vi "24_2.vi"() -> ()   [LabVIEW 2020]
uses:
  b6220058-4329-4b3d-852f-7dafbc0d4870.vi
panel:
  out "x-y":u32
  in  "Days":i32=100
  out "size":i32
  in  "Switch":bool
  in  "Input":string="nwneswnwnwsenwnwnwnwnwnwnwnwnwnenwnwnwnw\nseseswswseseswsesenwnwseseswsese\nswneeweneeneneeneeeeeneeeene\neswswnwswswwnwswswswswewswswswswswsw\nwwseneseeneseswwwseneseseneswseswese\nseseseswseseseseswnwswswneseseswsesesese\nnwnewwwwwswnwnwww\nneesenwwswseswswswnwsenwsesewseeeswse\nsweeneesweeswnweewseeneeneneswnw\nswseswseswswseseswseneswseswswsesesesese\nswneneneenenenenenenenenenenenwne\nswswswswswswswswswswswesenwseswswswse\nneeeenweneeneswene\nswwnenwsewwwswswwswwswweewwswwnw\nenewwnenwnenenenwnewnenenwnenenenwee\nnwwnwnwnwnwnwnwenewnwsenwwwwwnwswnw\neeenweeeesweeeneeseeeeswee\nwswwswseswwswswwwnww\nswenwwn..."
  in  "Input Test":string="sesenwnenenewseeswwswswwnenewsewsw\nneeenesenwnwwswnenewnwwsewnenwseswesw\nseswneswswsenwwnwse\nnwnwneseeswswnenewneswwnewseswneseene\nswweswneswnenwsewnwneneseenw\neesenwseswswnenwswnwnwsewwnwsene\nsewnenenenesenwsewnenwwwse\nwenwwweseeeweswwwnwwe\nwsweesenenewnwwnwsenewsenwwsesesenwne\nneeswseenwwswnwswswnw\nnenwswwsewswnenenewsenwsenwnesesenew\nenewnwewneswsewnwswenweswnenwsenwsw\nsweneswneswneneenwnewenewwneswswnese\nswwesenesewenwneswnwwneseswwne\nenesenwswwswneneswsenwnewswseenwsese\nwnwnesenesenenwwnenwsewesewsesesew\nnenewswnwewswnenesenwnesewesw\neneswnwswnwsenenwnwnwwseeswneewsenese\nneswnwewnwnwseenwseesewsenwsweewe\nwseweeenwnesenwwwswnew"
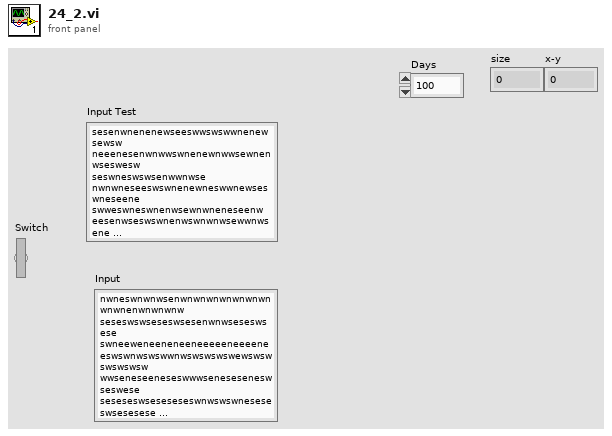
[diagram p1: front panel]
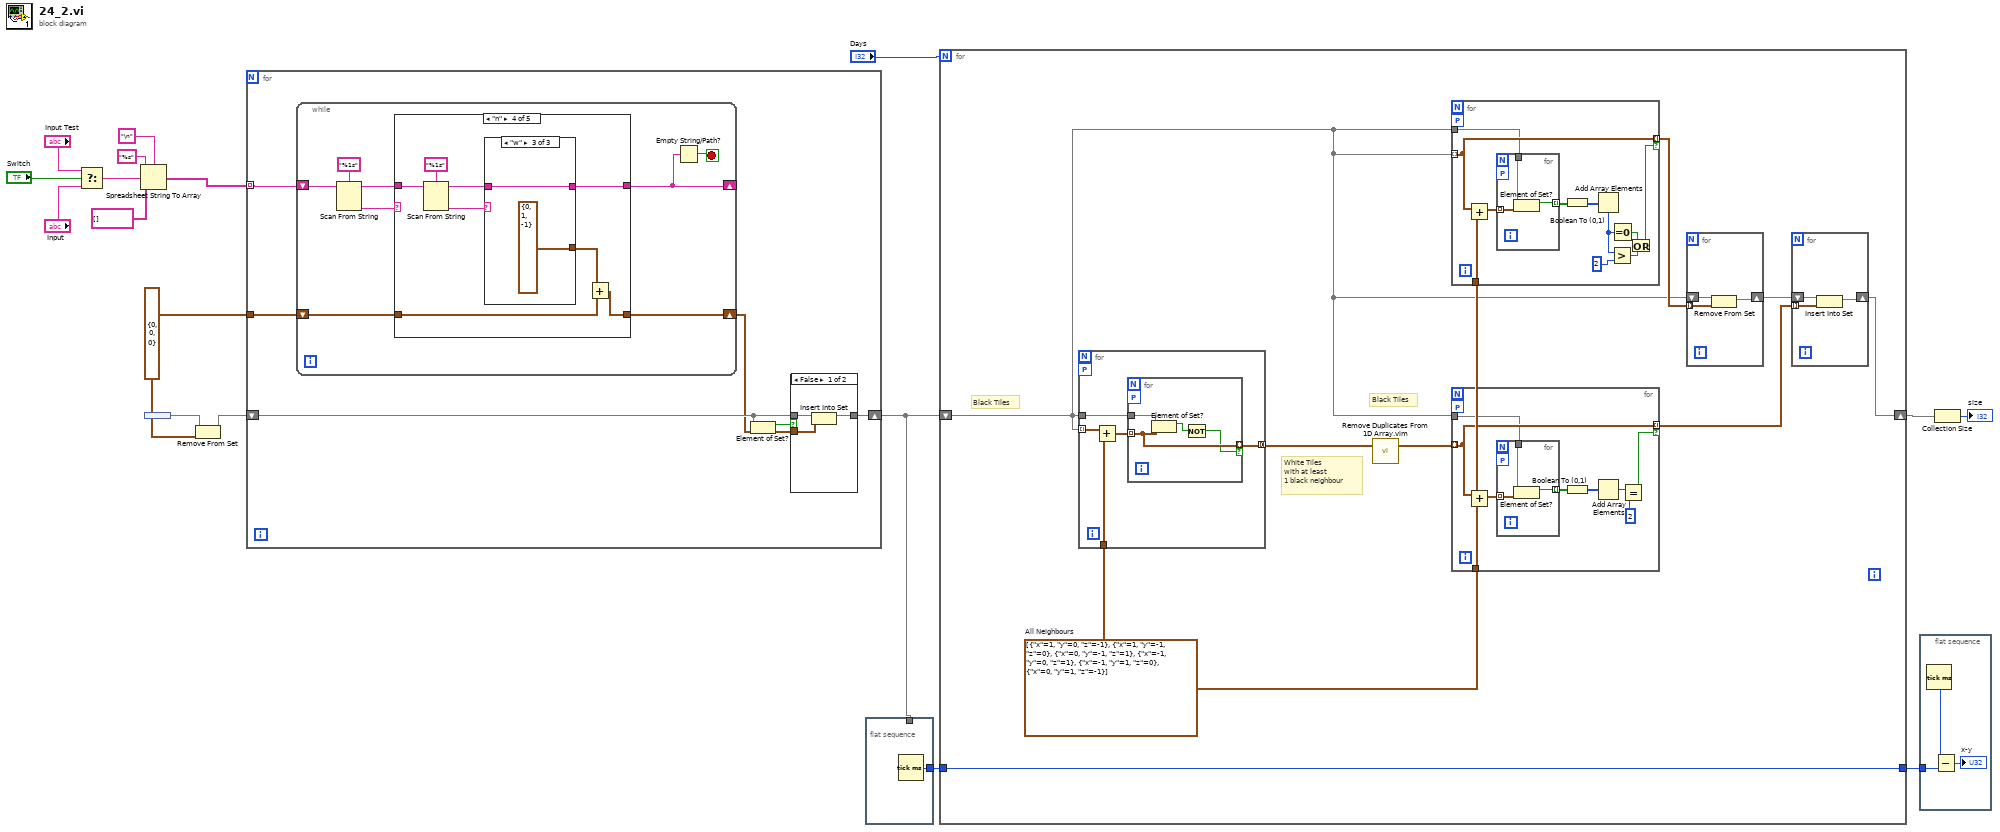
[diagram p0: block diagram]
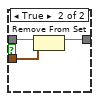
[diagram p2: hidden frame]
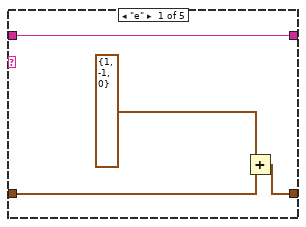
[diagram p3: hidden frame]
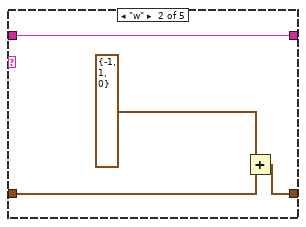
[diagram p4: hidden frame]
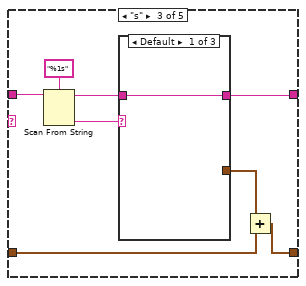
[diagram p5: hidden frame]
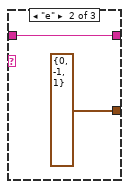
[diagram p6: hidden frame]
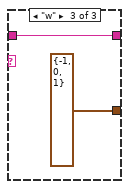
[diagram p7: hidden frame]
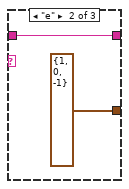
[diagram p9: hidden frame]
diagram:
  w7 = cluster{"x":i32, "y":i32, "z":i32} {"x"=0, "y"=0, "z"=0}
  n1 = Select(t="Input Test", s="Switch", f="Input") -> (s? t:f=w14:string)
  n2 = Spreadsheet String To Array(delimiter (Tab)="\n", format string="%s", spreadsheet string=w14, array type (2D Dbl)=string[] []) -> (array=w10:string[])
  n3 = node(w7) -> (w9:set{cluster{"x":i32, "y":i32, "z":i32}})
  n4 = Remove From Set(10:w7, 11:w9) -> (3:w8:set{cluster{"x":i32, "y":i32, "z":i32}})  [unwired: 1 out]
  n5 = for {
    tunnel: w10 -> [w23] mode=indexing
    tunnel: w7 -> [w22]
    shift-right: [w18] -> w1
    shift-left: w8 -> [w20]
    n6 = while {
      shift-right: [w32] -> _
      shift-left: w23 -> [w37]
      shift-right: [w30] -> w19
      shift-left: w22 -> [w31]
      stop <- w35 stop-if-true
      n7 = Scan From String(format string="%1s", input string=w37) -> (remaining string=w33:string, output 1=w34:string)  [unwired: 3 in, 2 out]
      n8 = case shown="\"n\"" w34 {
        tunnel: w33 -> [w41 w45 w49 w62 w73]
        tunnel: [w41 w45 w47 w60 w73] -> w32
        tunnel: w31 -> [w38 w42 w51 w64 w72]
        tunnel: [w39 w43 w52 w65 w72] -> w30
        frame "e" {
          n9 = Add(x=cluster{"x":i32, "y":i32, "z":i32} {"x"=1, "y"=-1, "z"=0}, y=w38) -> (x+y=w39:cluster{"x":i32, "y":i32, "z":i32})
        }
        frame "w" {
          n10 = Add(x=cluster{"x":i32, "y":i32, "z":i32} {"x"=-1, "y"=1, "z"=0}, y=w42) -> (x+y=w43:cluster{"x":i32, "y":i32, "z":i32})
        }
        frame "s" {
          n11 = Scan From String(format string="%1s", input string=w49) -> (remaining string=w48:string, output 1=w46:string)  [unwired: 3 in, 2 out]
          n12 = case shown="Default" w46 {
            tunnel: [_ cluster{"x":i32, "y":i32, "z":i32} {"x"=0, "y"=-1, "z"=1} cluster{"x":i32, "y":i32, "z":i32} {"x"=-1, "y"=0, "z"=1}] -> w53
            tunnel: [w54 w55 w57] -> w47
            tunnel: w48 -> [w54 w55 w57]
            frame Default {
            }
            frame "e" {
            }
            frame "w" {
            }
          }
          n13 = Add(x=w53, y=w51) -> (x+y=w52:cluster{"x":i32, "y":i32, "z":i32})
        }
        frame "n" {
          n14 = Scan From String(format string="%1s", input string=w62) -> (remaining string=w61:string, output 1=w59:string)  [unwired: 3 in, 2 out]
          n15 = case shown="\"w\"" w59 {
            tunnel: [_ cluster{"x":i32, "y":i32, "z":i32} {"x"=1, "y"=0, "z"=-1} cluster{"x":i32, "y":i32, "z":i32} {"x"=0, "y"=1, "z"=-1}] -> w66
            tunnel: [w67 w68 w70] -> w60
            tunnel: w61 -> [w67 w68 w70]
            frame Default {
            }
            frame "e" {
            }
            frame "w" {
            }
          }
          n16 = Add(x=w66, y=w64) -> (x+y=w65:cluster{"x":i32, "y":i32, "z":i32})
        }
        frame Default {
        }
      }
      n17 = Empty String/Path?(string/path=w32) -> (empty?=w35:bool)
    }
    n18 = Element of Set?(10:w19, 11:w20) -> (3:w21:bool)
    n19 = case shown="False" w21 {
      tunnel: w20 -> [w26 w29]
      tunnel: w19 -> [w24 w28]
      tunnel: [w25 w27] -> w18
      frame False {
        n20 = Insert Into Set(10:w24, 11:w26) -> (3:w25:set{cluster{"x":i32, "y":i32, "z":i32}})  [unwired: 1 out]
      }
      frame True {
        n21 = Remove From Set(10:w28, 11:w29) -> (3:w27:set{cluster{"x":i32, "y":i32, "z":i32}})  [unwired: 1 out]
      }
    }
  }
  n22 = flat-sequence {
    tunnel: [w74] -> w4
    tunnel: w1 -> [_]
    frame #0 {
      n23 = Tick Count (ms)() -> (millisecond timer value=w74:u32)
    }
  }
  n24 = for {
    N: "Days" -> [_]
    shift-right: [w81] -> w3
    shift-left: w1 -> [w77]
    tunnel: w4 -> [w78]
    tunnel: [w78] -> w2
    w80 = cluster{"x":i32, "y":i32, "z":i32}[] [{"x"=1, "y"=0, "z"=-1}, {"x"=1, "y"=-1, "z"=0}, {"x"=0, "y"=-1, "z"=1}, {"x"=-1, "y"=0, "z"=1}, {"x"=-1, "y"=1, "z"=0}, {"x"=0, "y"=1, "z"=-1}]  # All Neighbours
    # "Black Tiles"
    # "White Tiles\nwith at least\n1 black neighbour"
    # "Black Tiles"
    n25 = for {
      tunnel: w77 -> [w119] mode=indexing
      tunnel: w80 -> [w120]
      tunnel: [w116] -> w76 mode=concatenating
      tunnel: w77 -> [w118]
      workers-P: _ -> [_]
      n26 = Add(x=w119, y=w120) -> (x+y=w117:cluster{"x":i32, "y":i32, "z":i32}[])
      n27 = for {
        tunnel: w117 -> [w124] mode=indexing
        tunnel: [w124] -> w116 mode=indexing if=w122
        tunnel: w118 -> [w121]
        workers-P: _ -> [_]
        n28 = Element of Set?(10:w124, 11:w121) -> (3:w123:bool)
        n29 = Not(x=w123) -> (.not. x?=w122:bool)
      }
    }
    n30 = call "Remove Duplicates From 1D Array.vim"("array"=w76) -> ("array with duplicates removed"=w75:cluster{"x":i32, "y":i32, "z":i32}[])  [unwired: 10 in]
    n31 = for {
      tunnel: w77 -> [w91] mode=indexing
      tunnel: [w91] -> w79 mode=indexing if=w84
      tunnel: w77 -> [w89]
      tunnel: w80 -> [w90]
      workers-P: _ -> [_]
      n32 = Add(x=w91, y=w90) -> (x+y=w92:cluster{"x":i32, "y":i32, "z":i32}[])
      n33 = for {
        tunnel: w92 -> [w97] mode=indexing
        tunnel: [w95] -> w93 mode=indexing
        tunnel: w89 -> [w96]
        workers-P: _ -> [_]
        n34 = Element of Set?(10:w97, 11:w96) -> (3:w95:bool)
      }
      n35 = Boolean To (0,1)(Boolean=w93) -> (0, 1=w94:i16[])
      n36 = Add Array Elements(numeric array=w94) -> (sum=w85:i16)
      n37 = Greater?(x=w85, y=i16 2) -> (0:w88:bool)
      n38 = Equal To 0?(x=w85) -> (x = 0?=w87:bool)
      n39 = Or(x=w87, y=w88) -> (x .or. y?=w84:bool)
    }
    n40 = for {
      tunnel: w75 -> [w107] mode=indexing
      tunnel: [w107] -> w82 mode=indexing if=w112
      tunnel: w77 -> [w104]
      tunnel: w80 -> [w106]
      workers-P: _ -> [_]
      n41 = Add(x=w107, y=w106) -> (x+y=w108:cluster{"x":i32, "y":i32, "z":i32}[])
      n42 = for {
        tunnel: w108 -> [w115] mode=indexing
        tunnel: [w113] -> w109 mode=indexing
        tunnel: w104 -> [w114]
        workers-P: _ -> [_]
        n43 = Element of Set?(10:w115, 11:w114) -> (3:w113:bool)
      }
      n44 = Boolean To (0,1)(Boolean=w109) -> (0, 1=w110:i16[])
      n45 = Add Array Elements(numeric array=w110) -> (sum=w105:i16)
      n46 = Equal?(x=w105, y=i16 2) -> (x = y?=w112:bool)
    }
    n47 = for {
      shift-right: [w101] -> w83
      shift-left: w77 -> [w103]
      tunnel: w79 -> [w102] mode=indexing
      n48 = Remove From Set(10:w102, 11:w103) -> (3:w101:set{cluster{"x":i32, "y":i32, "z":i32}})  [unwired: 1 out]
    }
    n49 = for {
      shift-right: [w98] -> w81
      shift-left: w83 -> [w100]
      tunnel: w82 -> [w99] mode=indexing
      n50 = Insert Into Set(10:w99, 11:w100) -> (3:w98:set{cluster{"x":i32, "y":i32, "z":i32}})  [unwired: 1 out]
    }
  }
  n51 = flat-sequence {
    tunnel: w2 -> [w127]
    frame #0 {
      n52 = Tick Count (ms)() -> (millisecond timer value=w126:u32)
      n53 = Subtract(x=w126, y=w127) -> (x-y=→"x-y":u32)
    }
  }
  n54 = Collection Size(1:w3) -> (0:→"size":i32)
